vi "Set Dimming.vi"(7 "Position":u32, 8 "error in (no error)":errorcluster, 9 "Dimming Type":string, 10 "Dim Level":dbl format="%#_13g", 11 "Driver Test in":refnum<class "Driver Test.lvclass">) -> (0 "error out":errorcluster)   [LabVIEW 2015, in "Driver Test.lvclass"]
doc: "Set dim level based on recipe driven Dim Type."
uses:
  Driver Test.lvclass
  CBTF Applications/Driver Board Testing/Main/Application/Application/Class/typedefs/Instrument Selector -- Enum.ctl
  Classes/Instruments/Power Supply/Class/Power Supply.lvclass
  CBTF Applications/Driver Board Testing/Main/Application/Application/Class/Driver Board Test.lvclass
  Test Class/Test Class.lvclass
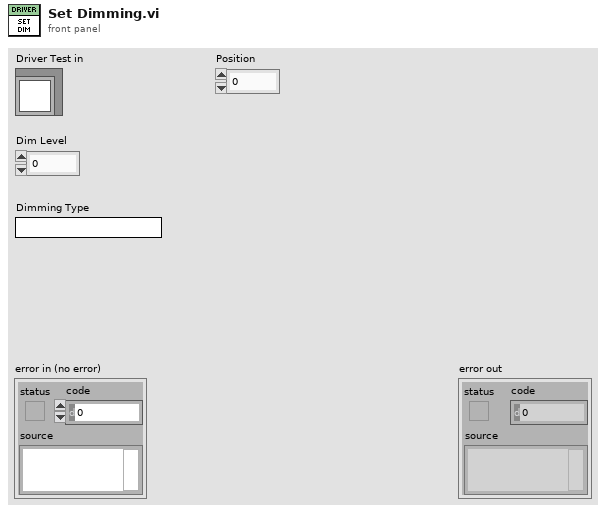
[diagram p1: front panel]
types:
  T1 = typedef "Driver Board Test.lvlib/Driver Board Test.lvclass/Instrument Selector -- Enum.ctl" = enum16{"ACPS1", "ACPS2", "DCPS1", "DCPS2", "DCPS3", "DCLoad1", "DCLoad2", "DPM1", "DPM2", "Switch1", "PXI1Slot2", "PXI1Slot3", "cDAQ1Mod5", "cDAQ1Mod6", "cDAQ1Mod7", "cDAQ1Mod8", "cDAQ1Mod1", "cDAQ1Mod2", "cDAQ1Mod3", "cDAQ1Mod4", "cDAQ2Mod1", "cDAQ2Mod2", "cDAQ2Mod3", "cDAQ2Mod4"}
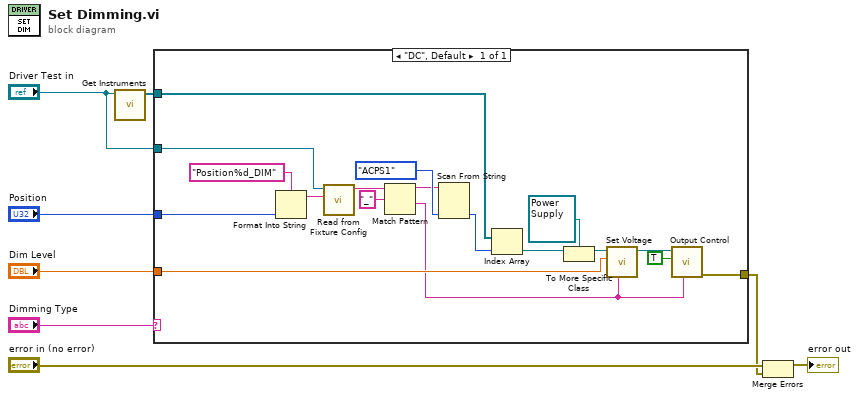
[diagram p0: block diagram]
diagram:
  n1 = call "Get Instruments.vi"("Test Class in"="Driver Test in") -> ("Instruments"=w1:refnum<class "Instrument.lvclass">[])  [unwired: 9 in, 1 out]
  n2 = case shown="\"DC\", Default" "Dimming Type" {
    tunnel: "Dim Level" -> [w25]
    tunnel: [w26] -> w2
    tunnel: "Position" -> [w13]
    tunnel: "Driver Test in" -> [w11]
    tunnel: w1 -> [w9]
    frame "DC", Default {
      n3 = Format Into String(format string="Position%d_DIM", w13) -> (resulting string=w12:string)  [unwired: 2 in, 1 out]
      n4 = call-dynamic "Read from Fixture Config.vi"("Key"=w12, "Test Class in"=w11) -> ("Instrument Info"=w10:string)  [unwired: 8 in, 1 out]
      n5 = Match Pattern(string=w10, regular expression="_") -> (before substring=w17:string, after substring=w15:string)  [unwired: 1 in, 2 out]
      n6 = Scan From String(input string=w17, default 1=Instrument_Selector_--_Enum."ACPS1" ("Instrument")) -> (output 1=w22:T1)  [unwired: 3 in, 3 out]
      n7 = Index Array(array=w9, index=w22) -> (element=w21:refnum<class "Instrument.lvclass">)
      n8 = To More Specific Class(target class=refnum<class "Power Supply.lvclass"> refnum ("Power Supply.lvlib:Power Supply.lvclass"), reference=w21) -> (specific class reference=w20:refnum<class "Power Supply.lvclass">)  [unwired: 1 in, 1 out]
      n9 = call-dynamic "Set Voltage.vi"("Channel (\"1\")"=w15, "Voltage (0.0 V)"=w25, "Acrobat Template in"=w20) -> ("Acrobat Template out"=w16:refnum<class "Power Supply.lvclass">)  [unwired: 7 in, 1 out]
      n10 = call-dynamic "Output Control.vi"("Channel (\"1\")"=w15, "Enabled"=TRUE, "Acrobat Template in"=w16) -> ("error out"=w26:errorcluster)  [unwired: 7 in, 1 out]
    }
  }
  n11 = Merge Errors("error in (no error)", w2) -> (→"error out":errorcluster)
